vi "Model Query.vi"(8 "error in (no error)":errorcluster, 11 "VISA resource name":refnum<visa-resource-name>) -> (0 "error out":errorcluster, 2 "Is DK242?":bool, 3 "VISA resource name out":refnum<visa-resource-name>)   [LabVIEW 2017, in "Digikrom DK24x.lvlib"]
doc: "IsDK242.vi - returns true if the device is a DK242, false if it is a DK240."
uses:
  Digikrom DK24x.lvlib
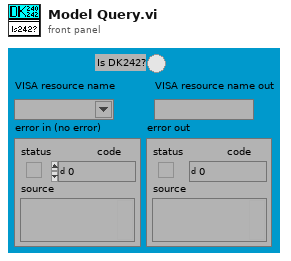
[diagram p1: front panel]
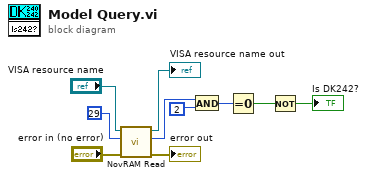
[diagram p0: block diagram]
diagram:
  n1 = call "NovRAM Read.vi"("error in (no error)"="error in (no error)", "NOVRAM ADDRESS"=29, "VISA resource name"="VISA resource name") -> ("error out"=→"error out":errorcluster, "WORD READ"=w1:u16, "VISA resource name out"=→"VISA resource name out":refnum<visa-resource-name>)  [unwired: 6 out]
  n2 = And(x=w1, y=u16 2) -> (x .and. y?=w9:u16)
  n3 = Equal To 0?(x=w9) -> (x = 0?=w8:bool)
  n4 = Not(x=w8) -> (.not. x?=→"Is DK242?":bool)
